vi "Pose_Exp.vi"(9 "TWIST":T1, 11 "POSE":T2) -> (3 "UpdatedPose":T2)   [LabVIEW 2019, in "Trajectory_Library.lvlib"]
doc: "Obtain a new Pose2d from a (constant curvature) velocity.\n\nSee <a href=\"https://file.tavsys.net/control/state-space-guide.pdf\"> Controls Engineering in the FIRST Robotics Competition</a> section on nonlinear pose estimation for derivation.\n\nThe twist is a change in pose in the robot's coordinate frame since the previous pose update. When the user runs exp() on the previous known field-relative pose with the argument being the twist, the user will receive the new field-relative pose.\n\n\"Exp\" represents the pose exponential, which is solving a differential equation moving the pose forward in time.\n\nPARAMETERS:\n--------------\n - POSE - current POSE data structure\n - TWIST - The change in pose in the robot's coordinate frame since the previous pose update. For example, if a non-holonomic robot moves forward 0.01 meters and changes angle by 0.5 degrees since the previous pose update, the twist would be Twist2d{0.01, 0.0, toRadians(0.5)}\n\nRETURNS:\n-----------\n- OUT POSE - The new pose of the robot."
uses:
  Trajectory_Library.lvlib
  POSE2D.ctl
  TRANSLATION2D.ctl
  ROTATION2D.ctl
  TWIST2D.ctl
  Util_CalcDist.vi
  Pose_TransformBy.vi
  Translation_RotateBy.vi
  Translation_Plus.vi
  Rotation_Plus.vi
  Pose_New_TRRO.vi
  Rotation_RotateBy.vi
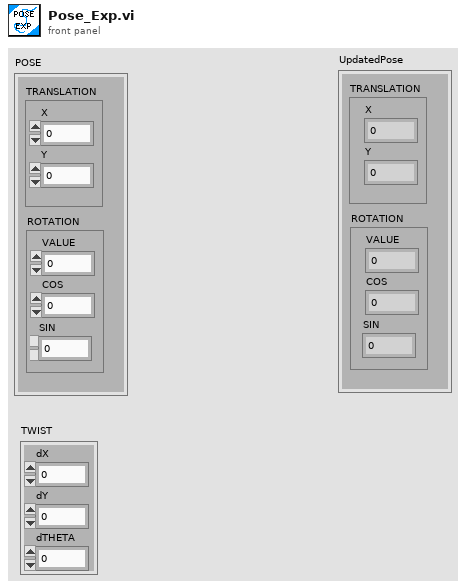
[diagram p1: front panel]
types:
  T1 = typedef "Trajectory_Library.lvlib/TWIST2D.ctl" = cluster{"dX":dbl, "dY":dbl, "dTHETA":dbl}
  T2 = typedef "Trajectory_Library.lvlib/POSE2D.ctl" = cluster{"TRANSLATION":T3, "ROTATION":T4}
  T3 = typedef "Trajectory_Library.lvlib/TRANSLATION2D.ctl" = cluster{"X":dbl, "Y":dbl}
  T4 = typedef "Trajectory_Library.lvlib/ROTATION2D.ctl" = cluster{"VALUE":dbl, "COS":dbl, "SIN":dbl}
  T5 = typedef "Trajectory_Library.lvlib/TRANSFORM2D.ctl" = cluster{"TRANSLATION":T3, "ROTATION":T4}
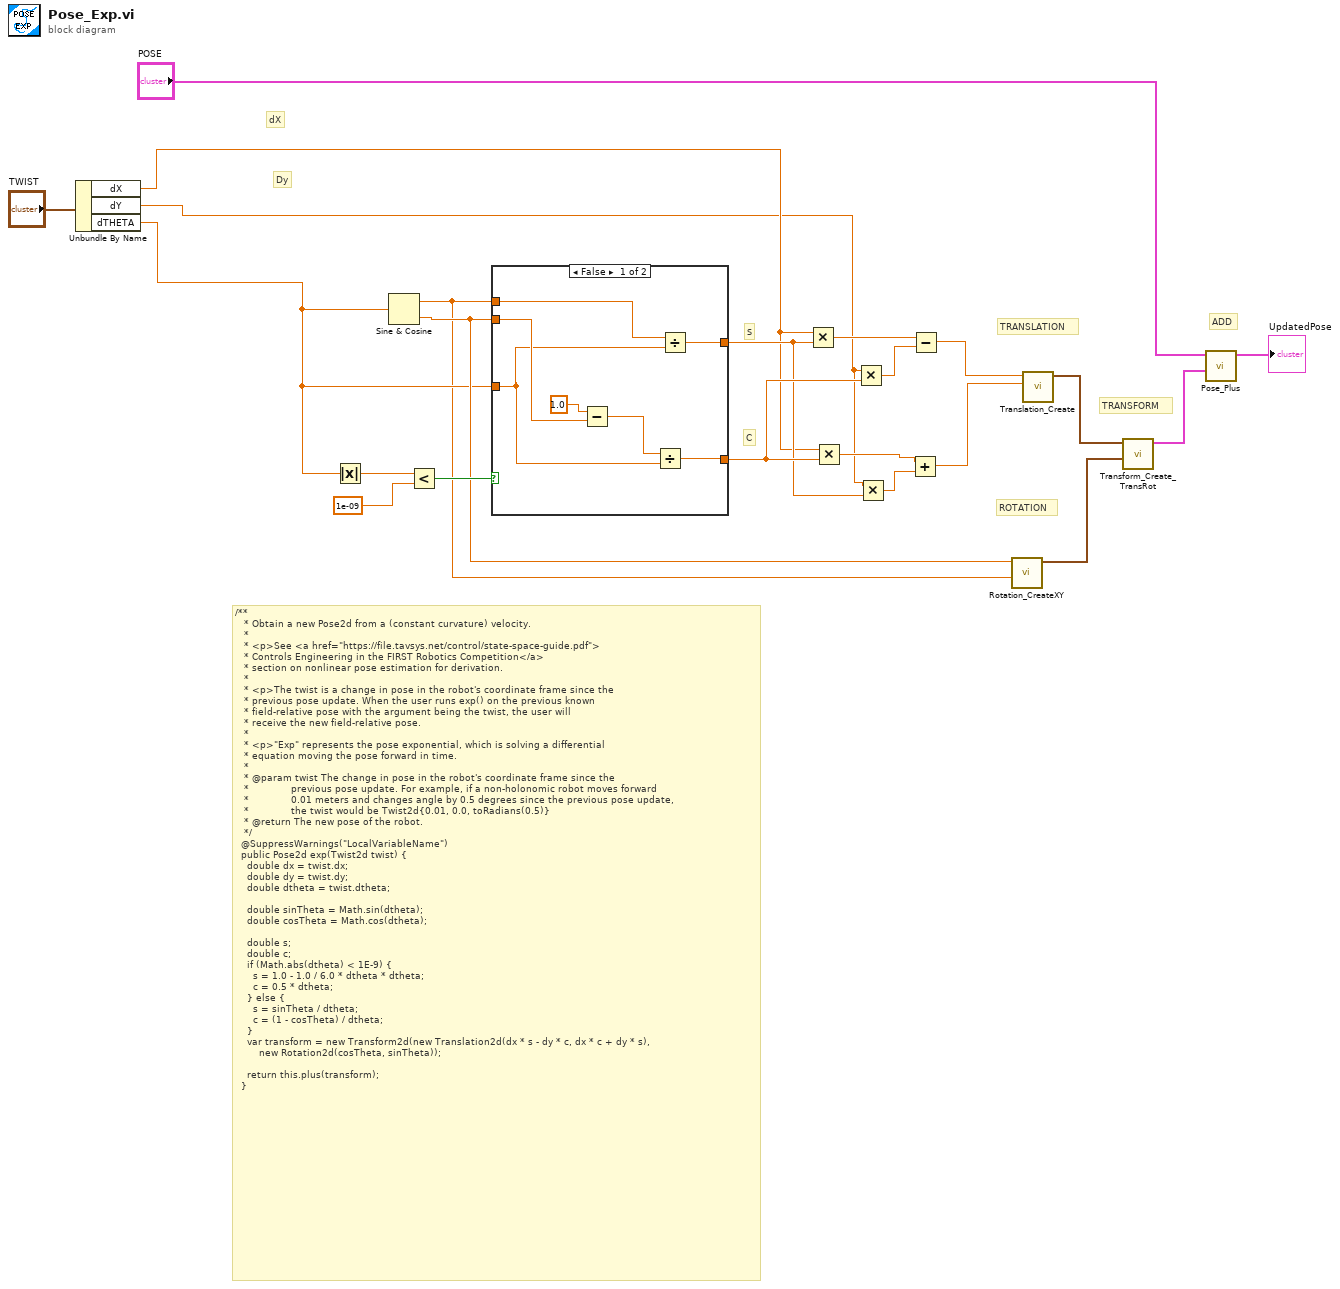
[diagram p0: block diagram]
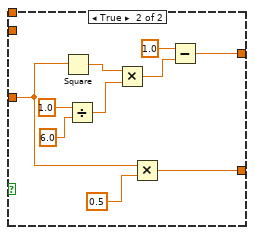
[diagram p2: hidden frame]
diagram:
  # "ADD"
  # "ROTATION"
  # "TRANSFORM"
  # "TRANSLATION"
  # "Dy"
  # "dX"
  # "C"
  # "S"
  # "/**\n   * Obtain a new Pose2d from a (constant curvature) velocity.\n   *\n   * <p>See <a href=\"https://file.tavsys.net/control/state-space-guide.pdf\">\n   * Controls Engineering in the FIRST Robotics Competition</a>\n   * section on nonlinear pose estimation for derivation.\n   *\n   * <p>The twist is a change in pose in the robot's coordinate frame since the\n   * previous pose update. When the user runs exp() on the previous known\n   * field-relative pose with the argument being the twist, the user will\n   * receive the new field-relative pose.\n   *\n   * <p>\"Exp\" represents the pose exponential, which is solving a differential\n   * equation moving the pose forward in time.\n   *\n   * @param twist The change in pose in the robot's coordinate frame since the\n   *              previous pose update. For example, if a non-holonomic robot moves forward\n   *              0.01 meters and changes angle by 0.5 degrees since the previous pose update,\n   *              the twist would be Twist2d{0.01, 0.0, toRadians(0.5)}\n   * @return The new pose of the robot.\n   */\n  @SuppressWarnings(\"LocalVariableName\")\n  public Pose2d exp(Twist2d twist) {\n    double dx = twist.dx;\n    double dy = twist.dy;\n    double dtheta = twist.dtheta;\n\n    double sinTheta = Math.sin(dtheta);\n    double cosTheta = Math.cos(dtheta);\n\n    double s;\n    double c;\n    if (Math.abs(dtheta) < 1E-9) {\n      s = 1.0 - 1.0 / 6.0 * dtheta * dtheta;\n      c = 0.5 * dtheta;\n    } else {\n      s = sinTheta / dtheta;\n      c = (1 - cosTheta) / dtheta;\n    }\n    var transform = new Transform2d(new Translation2d(dx * s - dy * c, dx * c + dy * s),\n        new Rotation2d(cosTheta, sinTheta));\n\n    return this.plus(transform);\n  }"
  n1 = Unbundle By Name("TWIST") -> ("dX"=w4:dbl, "dY"=w3:dbl, "dTHETA"=w2:dbl)
  n2 = Absolute Value(x=w2) -> (abs(x)=w21:dbl)
  n3 = Sine & Cosine(0:w2) -> (1:w1:dbl, 2:w11:dbl)
  n4 = Less?(x=w21, y=1e-09) -> (x < y?=w20:bool)
  n5 = case shown="False" w20 {
    tunnel: w2 -> [w23 w31]
    tunnel: [w28 w33] -> w16
    tunnel: [w25 w30] -> w19
    tunnel: w1 -> [w29 _]
    tunnel: w11 -> [w26 _]
    frame False {
      n6 = Subtract(x=1.0, y=w26) -> (x-y=w24:dbl)
      n7 = Divide(x=w24, y=w23) -> (x/y=w25:dbl)
      n8 = Divide(x=w29, y=w23) -> (x/y=w28:dbl)
    }
    frame True {
      n9 = Square(x=w31) -> (x^2=w36:dbl)
      n10 = Divide(x=1.0, y=6.0) -> (x/y=w35:dbl)
      n11 = Multiply(x=w36, y=w35) -> (x*y=w34:dbl)
      n12 = Multiply(x=w31, y=0.5) -> (x*y=w30:dbl)
      n13 = Subtract(x=1.0, y=w34) -> (x-y=w33:dbl)
    }
  }
  n14 = Multiply(x=w4, y=w16) -> (x*y=w18:dbl)
  n15 = Multiply(x=w4, y=w19) -> (x*y=w15:dbl)
  n16 = Multiply(x=w3, y=w19) -> (x*y=w17:dbl)
  n17 = Multiply(x=w3, y=w16) -> (x*y=w14:dbl)
  n18 = Add(x=w15, y=w14) -> (x+y=w12:dbl)
  n19 = Subtract(x=w18, y=w17) -> (x-y=w13:dbl)
  n20 = call "Rotation_CreateXY.vi"("Y or sine"=w1, "X or  cosine"=w11) -> ("ROTATION"=w10:T4)  [unwired: 9 in]
  n21 = call "Translation_Create.vi"("Y"=w12, "X"=w13) -> ("TRANSLATION"=w9:T3)  [unwired: 9 in]
  n22 = call "Transform_Create_TransRot.vi"("ROTATION"=w10, "TRANSLATION"=w9) -> ("TRANSFORM"=w8:T5)  [unwired: 9 in]
  n23 = call "Pose_Plus.vi"("other TRANSFORM"=w8, "in POSE"="POSE") -> ("out POSE"=→"UpdatedPose":T2)  [unwired: 9 in]
